vi "Wait.vi"(7 "Next Play":u32, 9 "YX Type":string, 11 "Maze 2.0.lvclass":refnum<class "SquareBattle.lvclass">) -> (1 "Success?":bool)   [LabVIEW 2014, in "SquareBattle.lvclass"]
uses:
  SquareBattle.lvclass
  SquareBattle.lvclass/SquareBattle.ctl
  Runner Cluster.ctl
  Runner/Runner.lvclass
panel:
  # "NOTICE - YOU MUST NOT REMOVE THIS NOTICE. PER THE FOLLOWING LICENSE, YOU MAY REPRODUCE THIS SOFTWARE PROVIDED YOU FOLLOW THE TERMS\nOF THE LICENSE.\n\n---BEGIN BSD LICENSE (http://opensource.org/licenses/BSD-2-Clause)---\nCopyright (c) 2015, Endigit, Inc. <robert@endigit.com>\nAll rights reserved.\n\nRedistribution and use in source and binary forms, with or without modification, are permitted provided that the following conditions are met:\n\n1. Redistributions of source code must retain the above copyright notice, this list of conditions and the following disclaimer.\n\n2. Redistributions in binary form must reproduce the above copyright notice, this list of conditions and the following disclaimer in the documentation and/or other \nmaterials provided with the distribution.\n\nTHIS SOFTWARE IS PROVIDED BY THE COPYRIGHT HOLDERS AND CONTRIBUTORS \"AS IS\" AND ANY EXPRESS OR IMPLIED WARRANTIES, INCLUDING, BUT NOT \nLIMITED TO, THE IMPLIED WARRANTIES OF MERCHANTABILITY AND FITNESS FOR A PARTICULAR PURPOSE ARE DISCLAIMED. IN NO EVENT SHALL THE COPYRIGHT \nHOLDER OR CONTRIBUTORS BE LIABLE FOR ANY DIRECT, INDIRECT, INCIDENTAL, SPECIAL, EXEMPLARY, OR CONSEQUENTIAL DAMAGES (INCLUDING, BUT NOT \nLIMITED TO, PROCUREMENT OF SUBSTITUTE GOODS OR SERVICES; LOSS OF USE, DATA, OR PROFITS; OR BUSINESS INTERRUPTION) HOWEVER CAUSED AND ON \nANY THEORY OF LIABILITY, WHETHER IN CONTRACT, STRICT LIABILITY, OR TORT (INCLUDING NEGLIGENCE OR OTHERWISE) ARISING IN ANY WAY OUT OF THE USE \nOF THIS SOFTWARE, EVEN IF ADVISED OF THE POSSIBILITY OF SUCH DAMAGE.\n---END BSD LICENSE---"
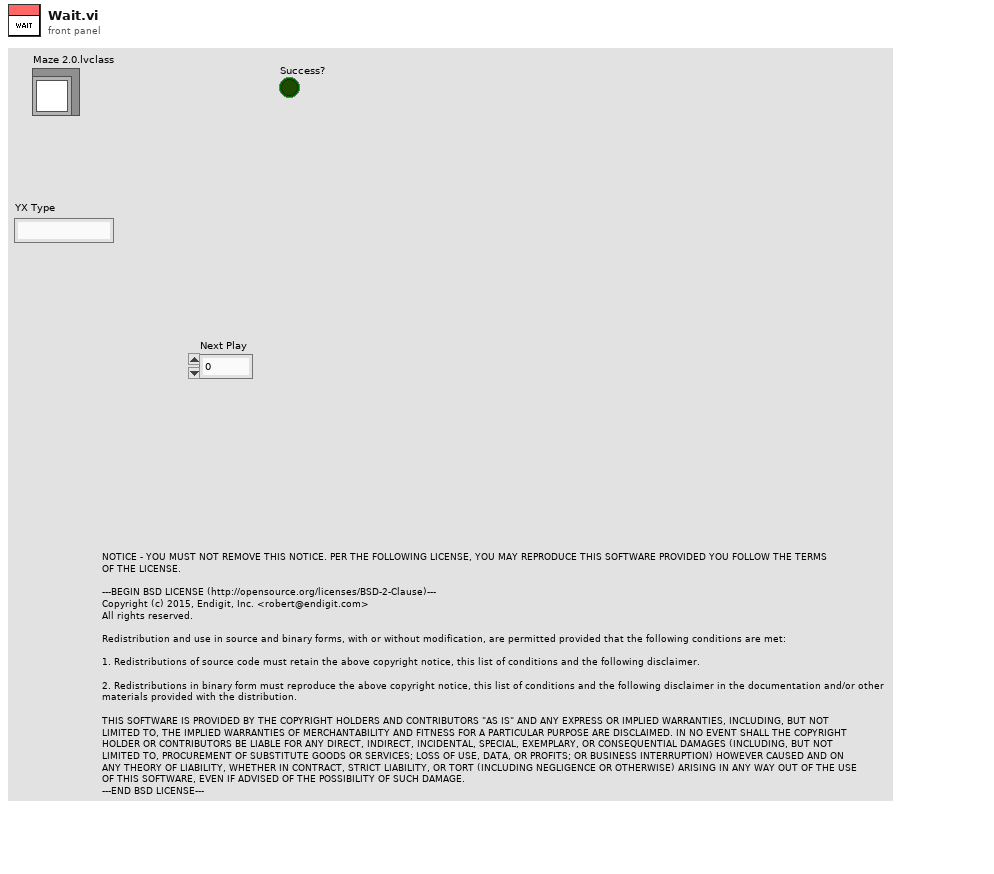
[diagram p1: front panel]
types:
  T1 = typedef "SquareBattle.lvclass/Runner Cluster.ctl" = cluster{"Attacked?":bool, "DVR":refnum<data-value>, "Team":i32, "Player":i32, "Wait":u32}
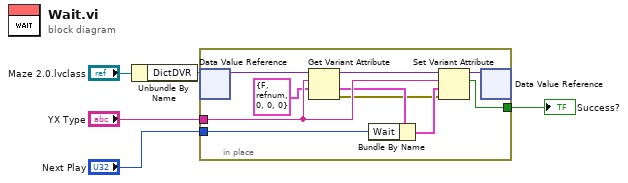
[diagram p0: block diagram]
diagram:
  n1 = Unbundle By Name("Maze 2.0.lvclass") -> ("DictDVR"=w4:refnum<data-value>)
  n2 = in-place {
    in-place-border: "YX Type" -> [w12]
    in-place-border: "Next Play" -> [w9]
    in-place-border: [w7] -> w1
    n3 = in-place-dvr #1(w4) -> (w15:variant)  [unwired: 1 out]
    n4 = Get Variant Attribute(Variant=w15, name=w12, default value (empty Variant)=T1 {"Attacked?"=FALSE, "DVR"=refnum, "Team"=0, "Player"=0, "Wait"=0} ("Cluster")) -> (duplicate Variant=w14:variant, value=w11:T1, error out=w6:errorcluster)  [unwired: 1 in, 1 out]
    n5 = Bundle By Name(cluster=w11, "Wait"=w9) -> (w10:T1)
    n6 = Set Variant Attribute(Variant=w14, name=w12, value=w10, error in=w6) -> (Variant out=w13:variant, replaced=w7:bool)  [unwired: 1 out]
    n7 = in-place-dvr #1(w13) -> ()  [unwired: 2 out]
  }
  "Success?" <- w1
